vi "Nattify - Align 1 Row of FP Controls.vi"(0 "controls":refnum<vi>[](array[refnum]), 1 "grid size":i32, 5 "top bound":i32, 11 "error in":errorcluster) -> (4 "max bottom":i32, 15 "error out":errorcluster)   [LabVIEW 2020]
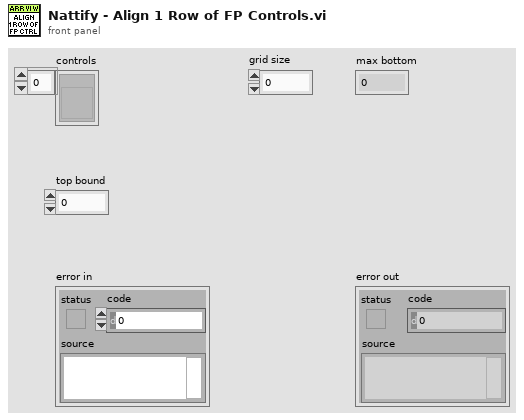
[diagram p1: front panel]
types:
  T1 = typedef "LVRectTypeDef.ctl" = cluster{"Left":i16, "Top":i16, "Right":i16, "Bottom":i16}
  T2 = cluster{"Left":i32, "Top":i32, "Right":i32, "Bottom":i32}
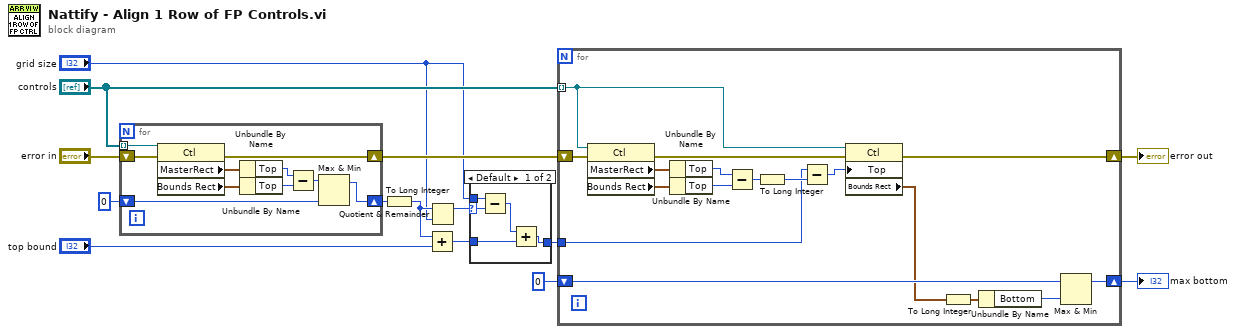
[diagram p0: block diagram]
diagram:
  n1 = for {
    shift-right: [w21] -> w11
    shift-left: "error in" -> [w22]
    shift-right: [w17] -> w8
    shift-left: i16 0 -> [w16]
    tunnel: "controls" -> [w15] mode=indexing
    n2 = property class="Ctl"(reference=w15, error in=w22) -> (error out=w21:errorcluster, "MasterRect"=w24:T1, "Bounds Rect"=w23:T1)  [unwired: 1 out]
    n3 = Unbundle By Name(w24) -> ("Top"=w19:i16)
    n4 = Unbundle By Name(w23) -> ("Top"=w20:i16)
    n5 = Subtract(x=w19, y=w20) -> (x-y=w18:i16)
    n6 = Max & Min(x=w18, y=w16) -> (max(x,y)=w17:i16)  [unwired: 1 out]
  }
  n7 = To Long Integer(number=w8) -> (32bit integer=w3:i32)
  n8 = Add(x=w3, y="top bound") -> (x+y=w6:i32)
  n9 = Quotient & Remainder(x=w3, y="grid size") -> (x-y*floor(x/y)=w7:i32)  [unwired: 1 out]
  n10 = case shown="Default" w7 {
    selector: w7 -> [w29 _]
    tunnel: "grid size" -> [w28 _]
    tunnel: [w27 w30] -> w4
    tunnel: w6 -> [w25 w30]
    frame Default {
      n11 = Subtract(x=w28, y=w29) -> (x-y=w26:i32)
      n12 = Add(x=w26, y=w25) -> (x+y=w27:i32)
    }
    frame 0 {
    }
  }
  n13 = for {
    tunnel: "controls" -> [w37] mode=indexing
    shift-right: [w43] -> w14
    shift-left: w11 -> [w42]
    shift-right: [w47] -> w13
    shift-left: 0 -> [w46]
    tunnel: w4 -> [w36]
    n14 = property class="Ctl"(reference=w37, error in=w42) -> (error out=w32:errorcluster, "MasterRect"=w41:T1, "Bounds Rect"=w40:T1)  [unwired: 1 out]
    n15 = Unbundle By Name(w41) -> ("Top"=w35:i16)
    n16 = Unbundle By Name(w40) -> ("Top"=w34:i16)
    n17 = Subtract(x=w35, y=w34) -> (x-y=w39:i16)
    n18 = To Long Integer(number=w39) -> (32bit integer=w38:i32)
    n19 = Subtract(x=w36, y=w38) -> (x-y=w33:i32)
    n20 = property class="Ctl"(reference=w37, error in=w32, "Top"=w33) -> (error out=w43:errorcluster, "Bounds Rect"=w31:T1)  [unwired: 1 out]
    n21 = To Long Integer(number=w31) -> (32bit integer=w44:T2)
    n22 = Unbundle By Name(w44) -> ("Bottom"=w45:i32)
    n23 = Max & Min(x=w46, y=w45) -> (max(x,y)=w47:i32)  [unwired: 1 out]
  }
  "max bottom" <- w13
  "error out" <- w14
